vi "List interesting control names.vi"(8 "Error in":errorcluster, 11 "Rules":T1[](array[typedef])) -> (0 "Error out":errorcluster, 3 "Relevant Controls":string[](array[string]))   [LabVIEW 2019, in "LSS.lvlib"]
doc: "This VI takes a pre-parsed list of rules and finds for which controls the property control engine must register for value change events.\n\n<b>Inputs:</b>\n<b>Rules</b> - Pre-parsed list of rules to search through.\n<b>Error In</b> - Standard Error In terminal.\n\n<b>Outputs:</b>\n<b>Relevent Controls</b> - List of controls that the property control engine must register for their value change events.\n<b>Error Out</b> - Standard Error out terminal."
uses:
  LSS.lvlib
  Controls/Rule.ctl
  Controls/Criteria.ctl
  Controls/Comparison Types.ctl
  Controls/Effects.ctl
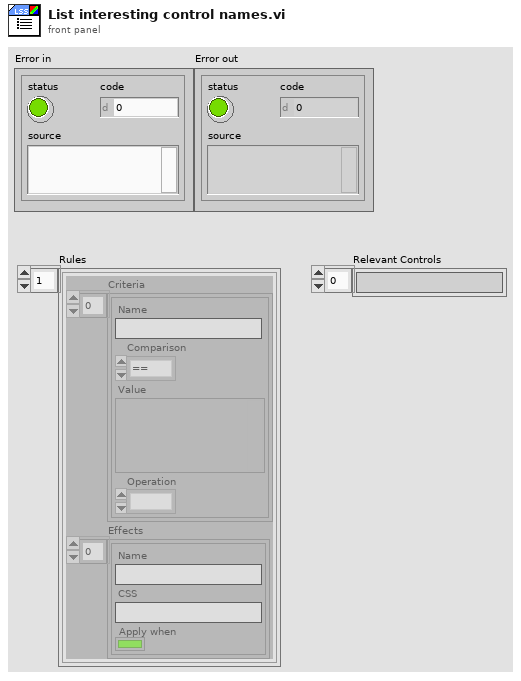
[diagram p1: front panel]
types:
  T1 = typedef "LSS.lvlib/Rule.ctl" = cluster{"Criteria":T2[], "Effects":T4[]}
  T2 = typedef "LSS.lvlib/Criteria.ctl" = cluster{"Name":string, "Comparison":T3, "Value":variant, "Operation":enum16{"Stack", "&&", "||"}}
  T3 = typedef "LSS.lvlib/Comparison Types.ctl" = enum16{"==", "!=", "<", ">", "<=", ">="}
  T4 = typedef "LSS.lvlib/Effects.ctl" = cluster{"Name":string, "CSS":string, "Apply when":bool}
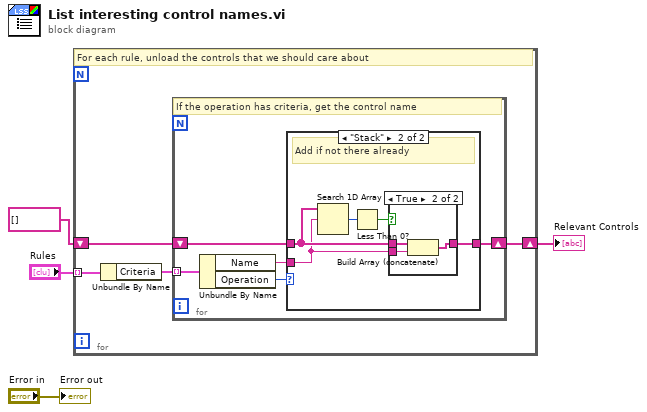
[diagram p0: block diagram]
diagram:
  n1 = for {
    tunnel: "Rules" -> [w8] mode=indexing
    shift-right: [w5] -> w1
    shift-left: string[] [] -> [w6]
    # "For each rule, unload the controls that we should care about"
    n2 = Unbundle By Name(w8) -> ("Criteria"=w7:T2[])
    n3 = for {
      tunnel: w7 -> [w13] mode=indexing
      shift-right: [w10] -> w5
      shift-left: w6 -> [w12]
      # "If the operation has criteria, get the control name"
      n4 = Unbundle By Name(w13) -> ("Name"=w11:string, "Operation"=w9:enum16{"Stack", "&&", "||"})
      n5 = case shown="\"Stack\"" w9 {
        tunnel: w12 -> [w14 w17]
        tunnel: w11 -> [_ w16]
        tunnel: [w14 w15] -> w10
        frame Default {
          # "No criteria"
        }
        frame "Stack" {
          # "Add if not there already"
          n6 = Search 1D Array(1D array=w17, element=w16) -> (index of element=w19:i32)  [unwired: 1 in]
          n7 = Less Than 0?(x=w19) -> (x < 0?=w18:bool)
          n8 = case shown="True" w18 {
            tunnel: w17 -> [w20 w23]
            tunnel: w16 -> [_ w22]
            tunnel: [w20 w21] -> w15
            frame False {
            }
            frame True {
              n9 = Build Array (concatenate)(w23, w22) -> (w21:string[])
            }
          }
        }
      }
    }
  }
  "Relevant Controls" <- w1
  "Error out" <- "Error in"
